vi "Write Current Ref.vi"(8 "error in (no error)":errorcluster, 10 "Current Ref":refnum<vi>, 11 "Abstract Power Supply in":refnum<class "Abstract Power Supply.lvclass">) -> (0 "error out":errorcluster, 3 "Abstract Power Supply out":refnum<class "Abstract Power Supply.lvclass">)   [LabVIEW 2013, in "Generic Power Supply.lvlib" / "Abstract Power Supply.lvclass"]
uses:
  Abstract Power Supply.lvclass
  Abstract Power Supply.lvclass/Abstract Power Supply.ctl
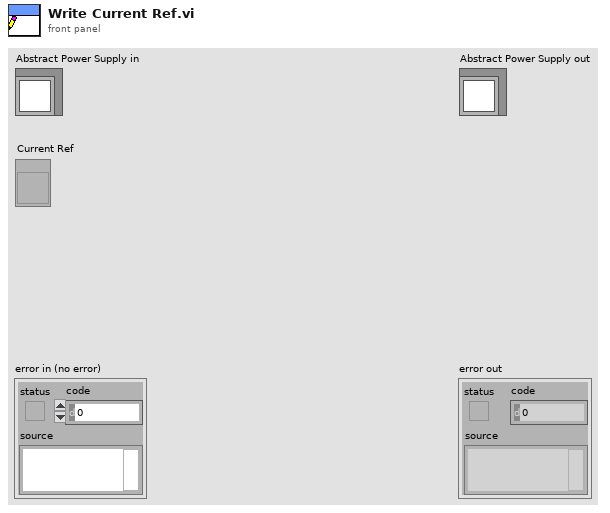
[diagram p1: front panel]
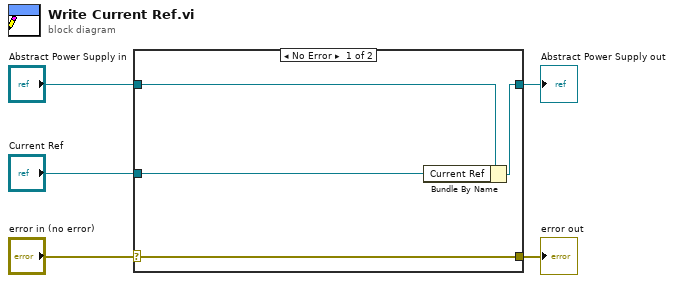
[diagram p0: block diagram]
diagram:
  n1 = case shown="No Error" "error in (no error)" {
    selector: "error in (no error)" -> [w9 w10]
    tunnel: [w9 w10] -> w4
    tunnel: [w7 w11] -> w2
    tunnel: "Abstract Power Supply in" -> [w8 w11]
    tunnel: "Current Ref" -> [w6 _]
    frame No Error {
      n2 = Bundle By Name(cluster=w8, "Current Ref"=w6) -> (w7:refnum<class "Abstract Power Supply.lvclass">)
    }
    frame Error {
    }
  }
  "error out" <- w4
  "Abstract Power Supply out" <- w2
